vi "Reorder channel.vi"(8 "error in (no error)":errorcluster, 11 "Channel Manager in":refnum<class "Channel Manager.lvclass">) -> (0 "error out":errorcluster, 3 "Channel Manager out":refnum<class "Channel Manager.lvclass">)   [LabVIEW 2018, in "Channel Manager.lvclass"]
uses:
  Channel Manager.lvclass
  Channel Manager.lvclass/Channel Manager.ctl
  Channel/Channel.lvclass/Channel.ctl
  Simulated_CCD_Camera/Simulated_CCD_Camera.lvclass
  Channel/Channel.lvclass
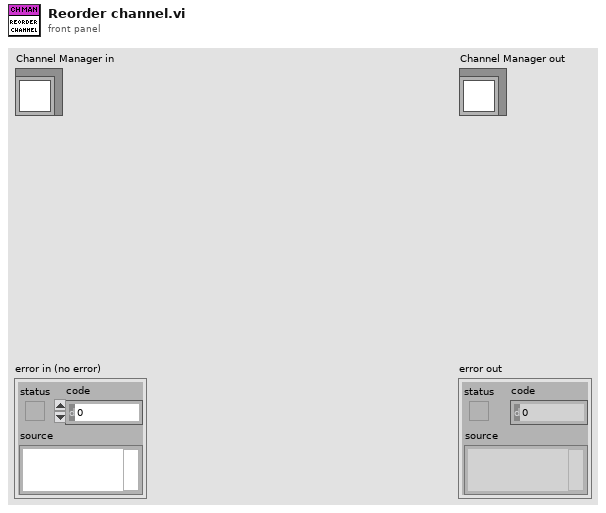
[diagram p1: front panel]
types:
  T1 = cluster{"CUBE_EXPOSURE_TIME":sgl, "CUBES_DONE":u16, "LAST_IMAGE_NAME":string, "DISK_SPACE":u16, "FRAMES_DONE":u16, "CCD_STATUS":string, "CURRENT_TEMPERATURE":i16, "TEMPERATURE_STATUS":string, "FRAME_EXPOSURE_TIME":u16, "CCD_ON_OFF":bool, "SERIAL_NUMBER":u16, "ACQUIRING":bool}
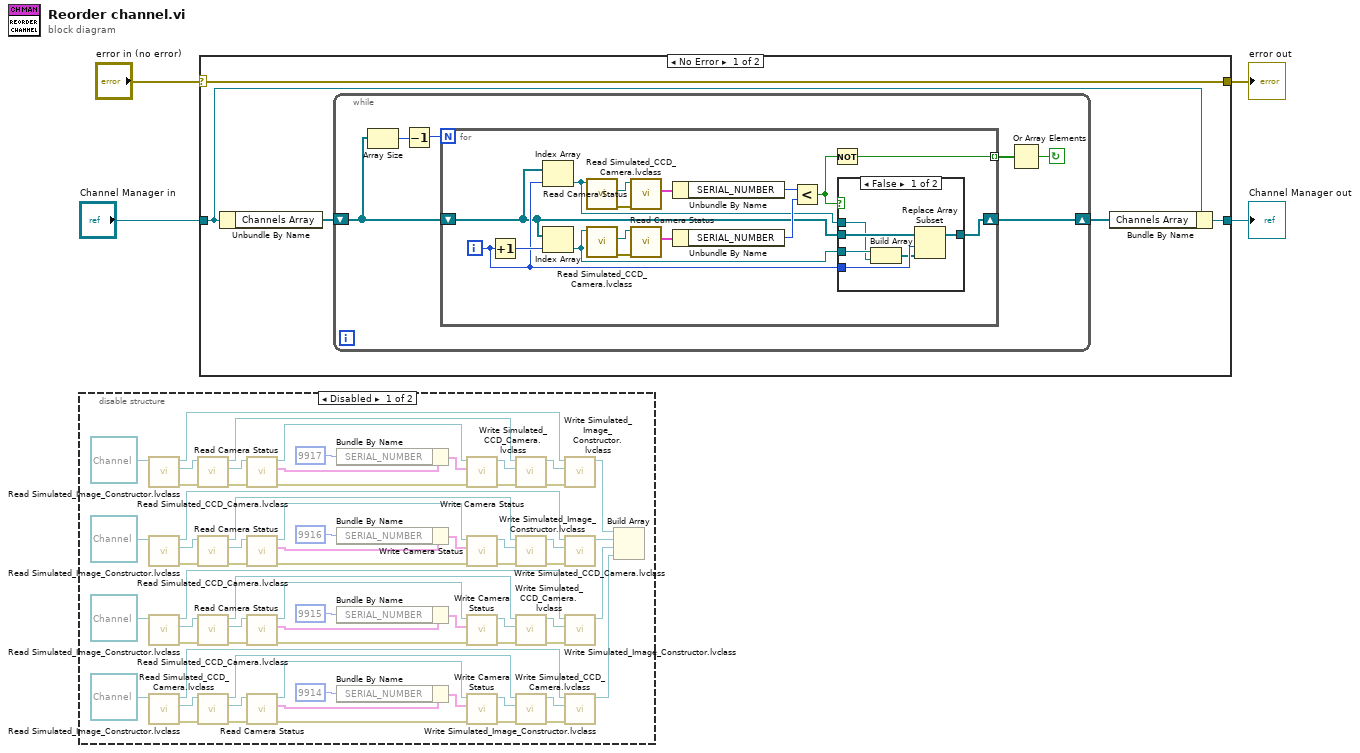
[diagram p0: block diagram]
diagram:
  n1 = disable-structure shown="Disabled" {
    frame Disabled {
      n2 = call "Read Simulated_Image_Constructor.lvclass.vi"("Channel in"=refnum<class "Channel.lvclass"> refnum) -> ("error out"=w66:errorcluster, "Simulated_Image_Constructor.lvclass"=w65:refnum<class "Simulated_Image_Constructor.lvclass">, "Channel out"=w18:refnum<class "Channel.lvclass">)  [unwired: 8 in]
      n3 = call "Read Simulated_Image_Constructor.lvclass.vi"("Channel in"=refnum<class "Channel.lvclass"> refnum) -> ("error out"=w59:errorcluster, "Simulated_Image_Constructor.lvclass"=w60:refnum<class "Simulated_Image_Constructor.lvclass">, "Channel out"=w15:refnum<class "Channel.lvclass">)  [unwired: 8 in]
      n4 = call "Read Simulated_Image_Constructor.lvclass.vi"("Channel in"=refnum<class "Channel.lvclass"> refnum) -> ("error out"=w46:errorcluster, "Simulated_Image_Constructor.lvclass"=w45:refnum<class "Simulated_Image_Constructor.lvclass">, "Channel out"=w12:refnum<class "Channel.lvclass">)  [unwired: 8 in]
      n5 = call "Read Simulated_Image_Constructor.lvclass.vi"("Channel in"=refnum<class "Channel.lvclass"> refnum) -> ("error out"=w39:errorcluster, "Simulated_Image_Constructor.lvclass"=w40:refnum<class "Simulated_Image_Constructor.lvclass">, "Channel out"=w9:refnum<class "Channel.lvclass">)  [unwired: 8 in]
      n6 = call "Read Simulated_CCD_Camera.lvclass.vi"("error in (no error)"=w66, "Image Constructor in"=w65) -> ("error out"=w67:errorcluster, "Simulated_CCD_Camera.lvclass"=w68:refnum<class "Simulated_CCD_Camera.lvclass">, "Image Constructor out"=w30:refnum<class "Simulated_Image_Constructor.lvclass">)  [unwired: 7 in]
      n7 = call "Read Simulated_CCD_Camera.lvclass.vi"("error in (no error)"=w59, "Image Constructor in"=w60) -> ("error out"=w58:errorcluster, "Simulated_CCD_Camera.lvclass"=w57:refnum<class "Simulated_CCD_Camera.lvclass">, "Image Constructor out"=w29:refnum<class "Simulated_Image_Constructor.lvclass">)  [unwired: 7 in]
      n8 = call "Read Simulated_CCD_Camera.lvclass.vi"("error in (no error)"=w46, "Image Constructor in"=w45) -> ("error out"=w47:errorcluster, "Simulated_CCD_Camera.lvclass"=w48:refnum<class "Simulated_CCD_Camera.lvclass">, "Image Constructor out"=w26:refnum<class "Simulated_Image_Constructor.lvclass">)  [unwired: 7 in]
      n9 = call "Read Simulated_CCD_Camera.lvclass.vi"("error in (no error)"=w39, "Image Constructor in"=w40) -> ("error out"=w38:errorcluster, "Simulated_CCD_Camera.lvclass"=w37:refnum<class "Simulated_CCD_Camera.lvclass">, "Image Constructor out"=w21:refnum<class "Simulated_Image_Constructor.lvclass">)  [unwired: 7 in]
      n10 = call "Read Camera Status.vi"("error in (no error)"=w67, "CCDCamera in"=w68) -> ("error out"=w70:errorcluster, "Camera Status"=w71:T1, "CCDCamera out"=w69:refnum<class "Simulated_CCD_Camera.lvclass">)  [unwired: 7 in]
      n11 = call "Read Camera Status.vi"("error in (no error)"=w58, "CCDCamera in"=w57) -> ("error out"=w55:errorcluster, "Camera Status"=w54:T1, "CCDCamera out"=w56:refnum<class "Simulated_CCD_Camera.lvclass">)  [unwired: 7 in]
      n12 = call "Read Camera Status.vi"("error in (no error)"=w47, "CCDCamera in"=w48) -> ("error out"=w50:errorcluster, "Camera Status"=w51:T1, "CCDCamera out"=w49:refnum<class "Simulated_CCD_Camera.lvclass">)  [unwired: 7 in]
      n13 = call "Read Camera Status.vi"("error in (no error)"=w38, "CCDCamera in"=w37) -> ("error out"=w35:errorcluster, "Camera Status"=w34:T1, "CCDCamera out"=w36:refnum<class "Simulated_CCD_Camera.lvclass">)  [unwired: 7 in]
      n14 = Bundle By Name(cluster=w71, "SERIAL_NUMBER"=u16 9917) -> (w72:T1)
      n15 = Bundle By Name(cluster=w54, "SERIAL_NUMBER"=u16 9916) -> (w53:T1)
      n16 = Bundle By Name(cluster=w51, "SERIAL_NUMBER"=u16 9915) -> (w52:T1)
      n17 = Bundle By Name(cluster=w34, "SERIAL_NUMBER"=u16 9914) -> (w33:T1)
      n18 = call "Write Camera Status.vi"("error in (no error)"=w70, "Camera Status"=w72, "CCDCamera in"=w69) -> ("error out"=w31:errorcluster, "CCDCamera out"=w32:refnum<class "Simulated_CCD_Camera.lvclass">)  [unwired: 7 in]
      n19 = call "Write Camera Status.vi"("error in (no error)"=w55, "Camera Status"=w53, "CCDCamera in"=w56) -> ("error out"=w27:errorcluster, "CCDCamera out"=w28:refnum<class "Simulated_CCD_Camera.lvclass">)  [unwired: 7 in]
      n20 = call "Write Camera Status.vi"("error in (no error)"=w50, "Camera Status"=w52, "CCDCamera in"=w49) -> ("error out"=w24:errorcluster, "CCDCamera out"=w25:refnum<class "Simulated_CCD_Camera.lvclass">)  [unwired: 7 in]
      n21 = call "Write Camera Status.vi"("error in (no error)"=w35, "Camera Status"=w33, "CCDCamera in"=w36) -> ("error out"=w23:errorcluster, "CCDCamera out"=w22:refnum<class "Simulated_CCD_Camera.lvclass">)  [unwired: 7 in]
      n22 = call "Write Simulated_CCD_Camera.lvclass.vi"("error in (no error)"=w31, "Simulated_CCD_Camera.lvclass"=w32, "Image Constructor in"=w30) -> ("error out"=w19:errorcluster, "Image Constructor out"=w20:refnum<class "Simulated_Image_Constructor.lvclass">)  [unwired: 7 in]
      n23 = call "Write Simulated_CCD_Camera.lvclass.vi"("error in (no error)"=w27, "Simulated_CCD_Camera.lvclass"=w28, "Image Constructor in"=w29) -> ("error out"=w17:errorcluster, "Image Constructor out"=w16:refnum<class "Simulated_Image_Constructor.lvclass">)  [unwired: 7 in]
      n24 = call "Write Simulated_CCD_Camera.lvclass.vi"("error in (no error)"=w24, "Simulated_CCD_Camera.lvclass"=w25, "Image Constructor in"=w26) -> ("error out"=w14:errorcluster, "Image Constructor out"=w13:refnum<class "Simulated_Image_Constructor.lvclass">)  [unwired: 7 in]
      n25 = call "Write Simulated_CCD_Camera.lvclass.vi"("error in (no error)"=w23, "Simulated_CCD_Camera.lvclass"=w22, "Image Constructor in"=w21) -> ("error out"=w11:errorcluster, "Image Constructor out"=w10:refnum<class "Simulated_Image_Constructor.lvclass">)  [unwired: 7 in]
      n26 = call "Write Simulated_Image_Constructor.lvclass.vi"("error in (no error)"=w19, "Simulated_Image_Constructor.lvclass"=w20, "Channel in"=w18) -> ("Channel out"=w8:refnum<class "Channel.lvclass">)  [unwired: 7 in, 1 out]
      n27 = call "Write Simulated_Image_Constructor.lvclass.vi"("error in (no error)"=w17, "Simulated_Image_Constructor.lvclass"=w16, "Channel in"=w15) -> ("Channel out"=w7:refnum<class "Channel.lvclass">)  [unwired: 7 in, 1 out]
      n28 = call "Write Simulated_Image_Constructor.lvclass.vi"("error in (no error)"=w14, "Simulated_Image_Constructor.lvclass"=w13, "Channel in"=w12) -> ("Channel out"=w6:refnum<class "Channel.lvclass">)  [unwired: 7 in, 1 out]
      n29 = call "Write Simulated_Image_Constructor.lvclass.vi"("error in (no error)"=w11, "Simulated_Image_Constructor.lvclass"=w10, "Channel in"=w9) -> ("Channel out"=w5:refnum<class "Channel.lvclass">)  [unwired: 7 in, 1 out]
      n30 = Build Array(w8, w7, w6, w5) -> ()  [unwired: 1 out]
    }
    frame Enabled {
    }
  }
  n31 = case shown="No Error" "error in (no error)" {
    selector: "error in (no error)" -> [w77 w108]
    tunnel: [w77 w108] -> w3
    tunnel: [w74 w107] -> w1
    tunnel: "Channel Manager in" -> [w76 w107]
    frame No Error {
      n32 = Unbundle By Name(w76) -> ("Channels Array"=w73:refnum<class "Channel.lvclass">[])
      n33 = while {
        shift-right: [w83] -> w75
        shift-left: w73 -> [w80]
        stop <- w78 continue-if-true
        n34 = Array Size(array=w80) -> (size(s)=w82:i32)
        n35 = Decrement(x=w82) -> (x-1=w81:i32)
        n36 = for {
          N: w81 -> [_]
          shift-right: [w95] -> w83
          shift-left: w80 -> [w94]
          tunnel: [w90] -> w79 mode=indexing
          i -> [w96]
          n37 = Increment(x=w96) -> (x+1=w99:i32)
          n38 = Index Array(array=w94, index=w96) -> (element=w84:refnum<class "Channel.lvclass">)
          n39 = Index Array(array=w94, index=w99) -> (element=w85:refnum<class "Channel.lvclass">)
          n40 = call "Read Simulated_CCD_Camera.lvclass.vi"("Channel in"=w84) -> ("error out"=w88:errorcluster, "Simulated_CCD_Camera.lvclass"=w89:refnum<class "Simulated_CCD_Camera.lvclass">)  [unwired: 8 in, 1 out]
          n41 = call "Read Simulated_CCD_Camera.lvclass.vi"("Channel in"=w85) -> ("error out"=w86:errorcluster, "Simulated_CCD_Camera.lvclass"=w87:refnum<class "Simulated_CCD_Camera.lvclass">)  [unwired: 8 in, 1 out]
          n42 = call "Read Camera Status.vi"("error in (no error)"=w88, "CCDCamera in"=w89) -> ("Camera Status"=w92:T1)  [unwired: 7 in, 2 out]
          n43 = call "Read Camera Status.vi"("error in (no error)"=w86, "CCDCamera in"=w87) -> ("Camera Status"=w93:T1)  [unwired: 7 in, 2 out]
          n44 = Unbundle By Name(w92) -> ("SERIAL_NUMBER"=w98:u16)
          n45 = Unbundle By Name(w93) -> ("SERIAL_NUMBER"=w97:u16)
          n46 = Less?(x=w98, y=w97) -> (x < y?=w91:bool)
          n47 = Not(x=w91) -> (.not. x?=w90:bool)
          n48 = case shown="False" w91 {
            tunnel: w94 -> [w105 w106]
            tunnel: w96 -> [w104 _]
            tunnel: [w103 w106] -> w95
            tunnel: w85 -> [w102 _]
            tunnel: w84 -> [w101 _]
            frame False {
              n49 = Build Array(w102, w101) -> (w100:refnum<class "Channel.lvclass">[])
              n50 = Replace Array Subset(array=w105, new element=w100, index=w104) -> (w103:refnum<class "Channel.lvclass">[])
            }
            frame True {
            }
          }
        }
        n51 = Or Array Elements(Boolean array=w79) -> (logical OR=w78:bool)
      }
      n52 = Bundle By Name(cluster=w76, "Channels Array"=w75) -> (w74:refnum<class "Channel Manager.lvclass">)
    }
    frame Error {
    }
  }
  "error out" <- w3
  "Channel Manager out" <- w1
